vi "CRYProject Editor Global.vi"() -> ()   [LabVIEW 2013]
uses:
  CRYSystem/Typedef Control/CRYTS.ctl
  CRYSystem/Typedef Control/CRYStep.ctl
  CRYSystem/Typedef Control/CRYProjectViewCluster.ctl
  CRYSystem/Typedef Control/CRYHardware.ctl
  CRYSystem/Typedef Control/CRYHardware Channel Info.ctl
panel:
  in  "bProjectLoading Failed":bool
  in  "SubSequenceLanguage":T1(ring)
  in  "SequenceInsertTreeIndex":i32
  in  "SequenceInsert":bool
  in  "G_Calibration Step path":path
  in  "G_Audi Interface Step path":path
  in  "SoundCard Step Backup":T2={"No.VI"=0, "Category"="", "StepName"="", "Seq setup flattened"="", "Comment"="", "Steps config."=[], "Jump config"=[], "Start"=0.0, "Increment"=0.0, "Name"="Pa", "Unit"="Pa", "Y data"=1, "Y prefix"="", "Y dB ref"=1.0, "Y unit"="", "Repeat State Array"=[]} {"Repeat State Array"."Start" format="%#_5g"; "Y dB ref" format="%.1f"; "Y data" items=["dB", "Lin"]; "Start" format="%#_5g"}
  in  "Calibration Step Backup":T2={"No.VI"=0, "Category"="", "StepName"="", "Seq setup flattened"="", "Comment"="", "Steps config."=[], "Jump config"=[], "Start"=0.0, "Increment"=0.0, "Name"="Pa", "Unit"="Pa", "Y data"=1, "Y prefix"="", "Y dB ref"=1.0, "Y unit"="", "Repeat State Array"=[]} {"Repeat State Array"."Start" format="%#_5g"; "Y dB ref" format="%.1f"; "Y data" items=["dB", "Lin"]; "Start" format="%#_5g"}
  in  "Calibration Step VI No":i32
  in  "SoundCard Step VI No":i32
  in  "SoundCard":T3={"Name"="", "Analog I/O"=0, "Digital I/O"=0, "Channels"=2, "Dig Dev ID"=1, "N ports"=3, "Interface"=0, "Dig I/O Ports"=[{"port #"=1, "width"=8, "direction"=0}, {"port #"=2, "width"=8, "direction"=0}, {"port #"=3, "width"=8, "direction"=0}], "Interf settings"=[], "N interfs"=3, "udev SNs"=[], "udev enable"=FALSE, "Channel Array"=[], "Cal sequence"="", "SelectedIn"=0, "SelectedOut"=0, "SelectedTab"=0, "State"=FALSE, "Help"="", "Advanced"=FALSE, "In Audio Driver"=0, "Out Audio Driver"=0} {"Channel Array"."Coupling" items=["Default"=-1, "RSE"=10083, "NRSE"=10078, "Differential"=10106, "Pseudodifferential"=12529]; "Channel Array"."term config" items=["Default"=-1, "RSE"=10083, "NRSE"=10078, "Differential"=10106, "Pseudodifferential"=12529]; "Channel Array"."Anti-aliasing Factor (%fs)" format="%.2f"}
  in  "Calibration Step":T2={"No.VI"=0, "Category"="", "StepName"="", "Seq setup flattened"="", "Comment"="", "Steps config."=[], "Jump config"=[], "Start"=0.0, "Increment"=0.0, "Name"="Pa", "Unit"="Pa", "Y data"=1, "Y prefix"="", "Y dB ref"=1.0, "Y unit"="", "Repeat State Array"=[]} {"Repeat State Array"."Start" format="%#_5g"; "Y dB ref" format="%.1f"; "Y data" items=["dB", "Lin"]; "Start" format="%#_5g"}
  in  "SoundCard Step":T2={"No.VI"=0, "Category"="", "StepName"="", "Seq setup flattened"="", "Comment"="", "Steps config."=[], "Jump config"=[], "Start"=0.0, "Increment"=0.0, "Name"="Pa", "Unit"="Pa", "Y data"=1, "Y prefix"="", "Y dB ref"=1.0, "Y unit"="", "Repeat State Array"=[]} {"Repeat State Array"."Start" format="%#_5g"; "Y dB ref" format="%.1f"; "Y data" items=["dB", "Lin"]; "Start" format="%#_5g"}
  in  "Add Step":refnum<vi>
  in  "Expand/Collapse Btn":refnum<vi>
  in  "TS Tree1":refnum<vi>
  in  "Property seq":refnum<vi>
  in  "Property step":refnum<vi>
  in  "Remove":refnum<vi>
  in  "Move Up":refnum<vi>
  in  "Move Down":refnum<vi>
  in  "TS Name":refnum<vi>
  in  "Expand/Collapse":bool
  in  "ConfigureShow":bool
  in  "Sequence Index for Calibration":i32
  in  "Sequence Index for Hardware":i32
  in  "ProjectViewCluster Array":T5[](array[typedef])
  in  "bProjectChanged":bool
  in  "bProjectLoaded":bool
  in  "cMsgProject":T6
  in  "previous cursor ID":refnum<k1>
  in  "sWorkAction":string
  in  "New Sequence Number":u16
  in  "PathLog":path
  in  "TS Array":T7 {"Steps"."Repeat State Array"."Start" format="%#_5g"; "Steps"."Y dB ref" format="%.1f"; "Steps"."Y data" items=["dB", "Lin"]; "Steps"."Start" format="%#_5g"}
  in  "Display Step No":i32
  in  "Project Open Mode":bool
  in  "Project Exist?":bool
  in  "ExitStateVal":u8
  in  "ScrollStateFlg":bool
  in  "ScrollStateVal":u8
  in  "Calibration TS Array":T7 {"Steps"."Repeat State Array"."Start" format="%#_5g"; "Steps"."Y dB ref" format="%.1f"; "Steps"."Y data" items=["dB", "Lin"]; "Steps"."Start" format="%#_5g"}
  in  "step ID Max":i16
  in  "TS Edit Info":cluster{"In Channel":u16, "Out Channel":u16}
  in  "AddStepsVI":refnum<vi>
  in  "ProjectView VI":refnum<vi>
  in  "AddStepCluster":T8
  in  "Task Sequence NameRef":refnum<vi>
  in  "Default TS Name":string
  in  "AddStepContent":T9(array[cluster])
  in  "SelectTreeStepNumber":i32
  in  "Step Setup VI No":i32
  # "Curves Array"
  # "max value"
  # "Selected Curves Array"
  # "old step edit num"
  # "current edit step"
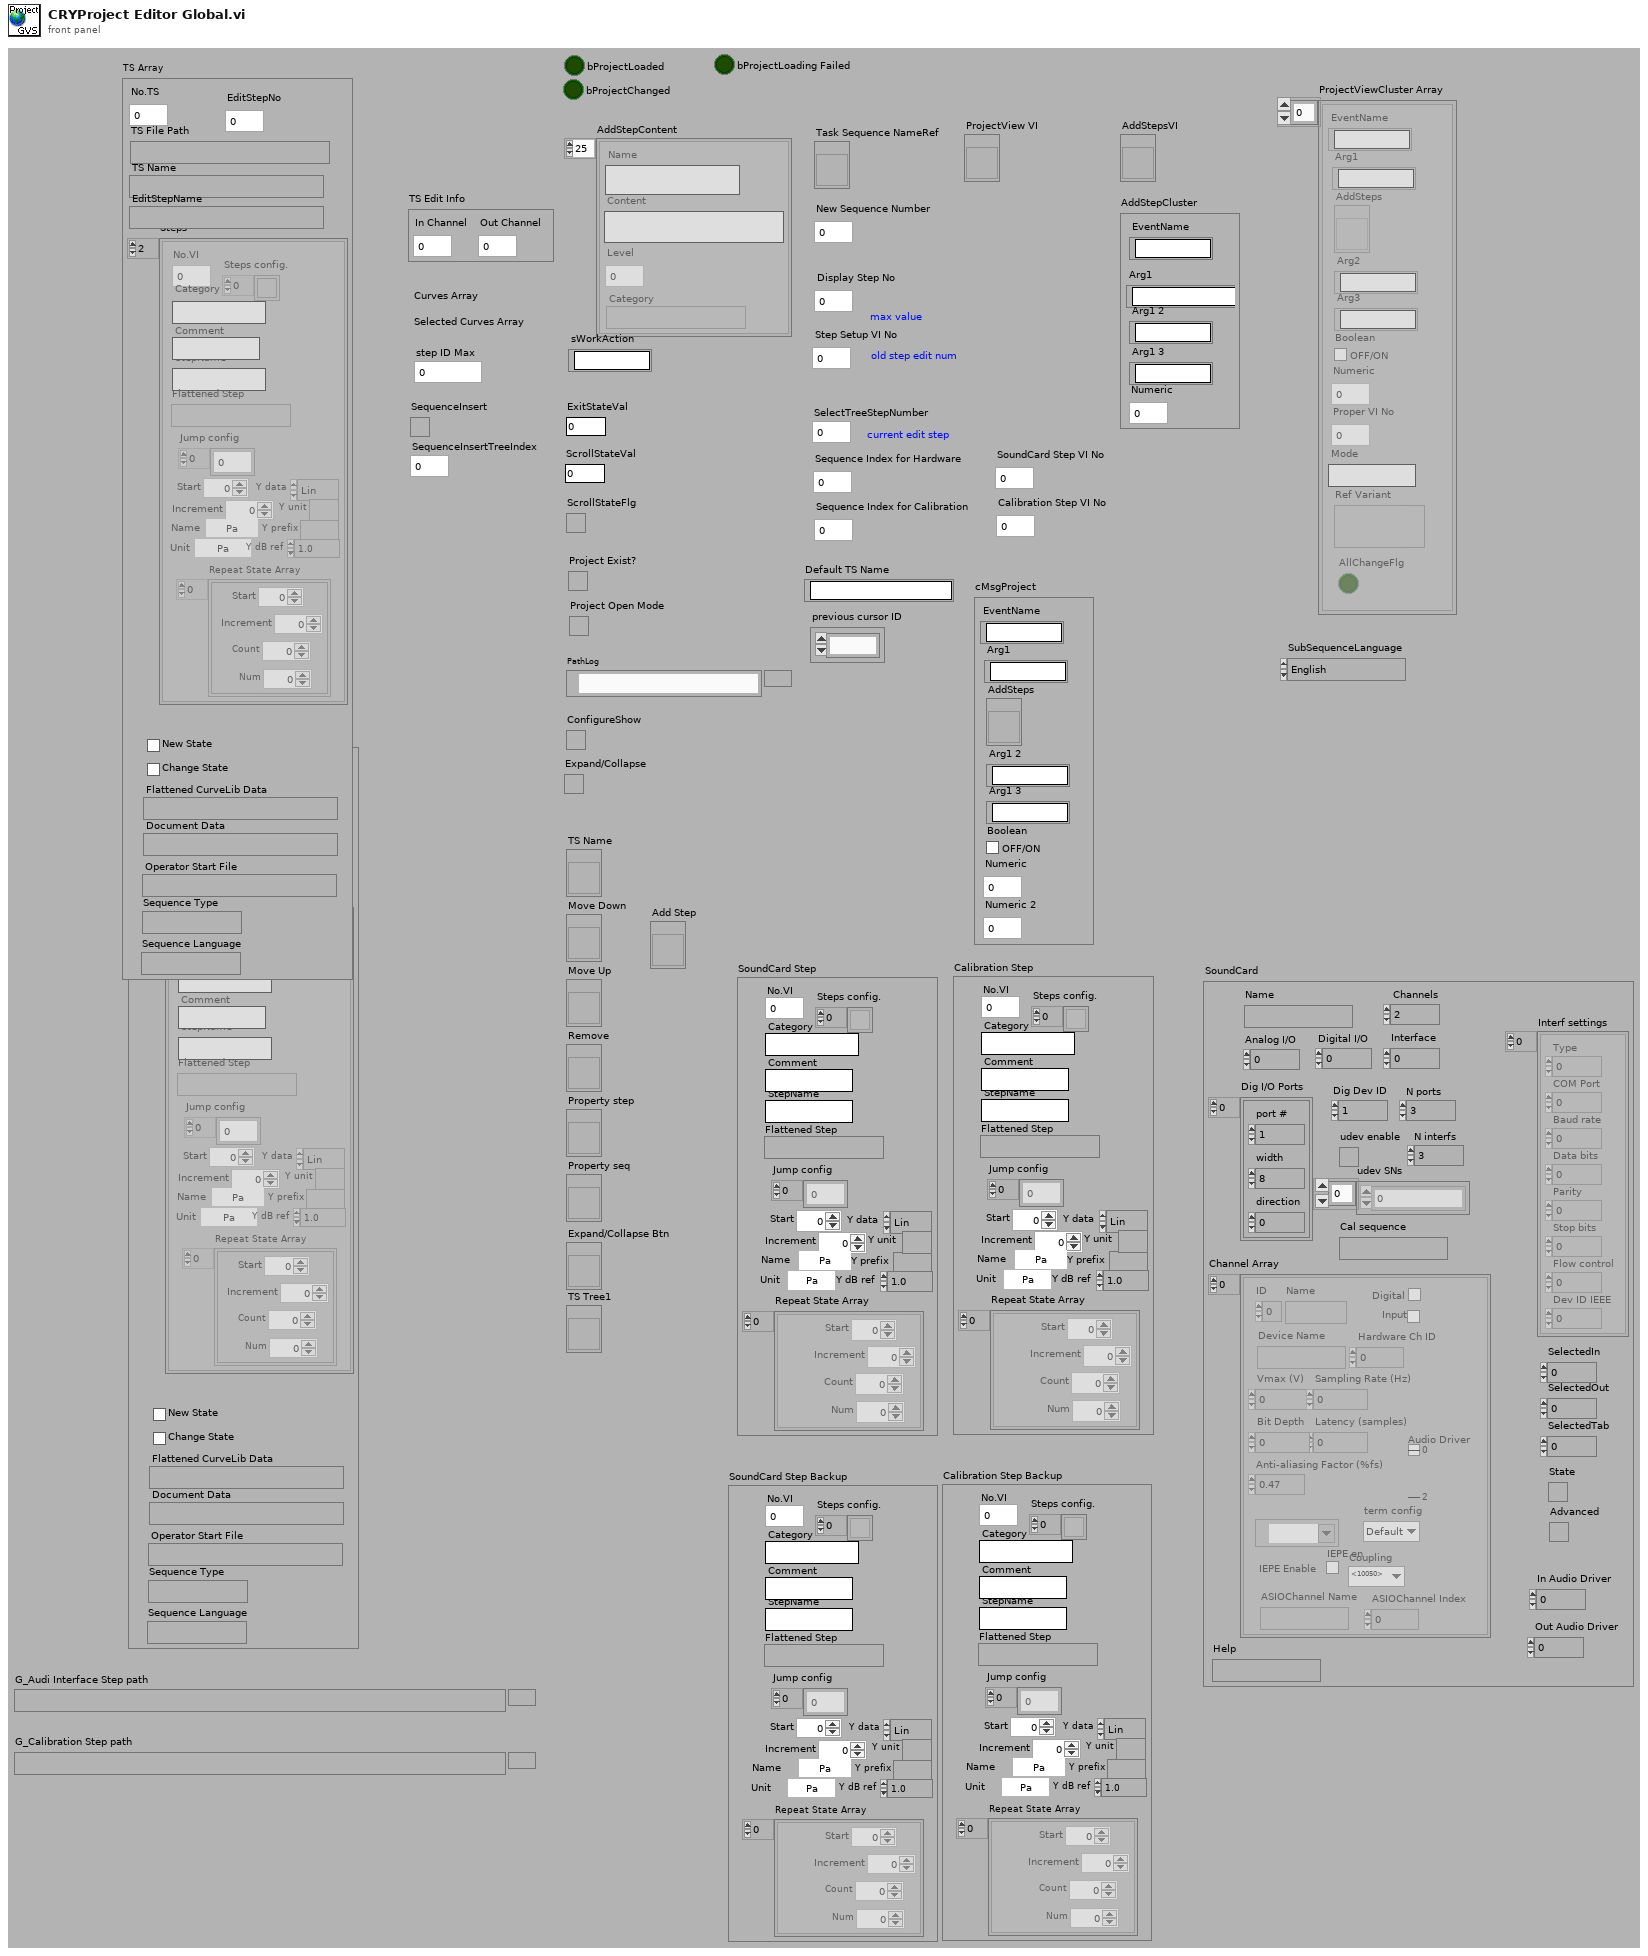
[diagram p1: front panel]
types:
  T1 = enum32{"English", "Chinese", "Korean", "Japanese", "Russian", "Chinese traditional"}
  T2 = typedef "CRYStep.ctl" = cluster{"No.VI":i32, "Category":string, "StepName":string, "Seq setup flattened":string, "Comment":string, "Steps config.":bool[], "Jump config":i32[], "Start":dbl, "Increment":dbl, "Name":string, "Unit":string, "Y data":u16, "Y prefix":string, "Y dB ref":dbl, "Y unit":string, "Repeat State Array":cluster{"Start":dbl, "Increment":dbl, "Count":i32, "Num":i32}[]}
  T3 = typedef "CRYHardware.ctl" = cluster{"Name":string, "Analog I/O":u16, "Digital I/O":u16, "Channels":u8, "Dig Dev ID":u8, "N ports":u8, "Interface":u32, "Dig I/O Ports":cluster{"port #":i16, "width":i16, "direction":i32}[], "Interf settings":cluster{"Type":u16, "COM Port":u8, "Baud rate":u32, "Data bits":u32, "Parity":u16, "Stop bits":u16, "Flow control":u16, "Dev ID IEEE":u8}[], "N interfs":i32, "udev SNs":i16[], "udev enable":bool, "Channel Array":T4[], "Cal sequence":string, "SelectedIn":u16, "SelectedOut":u16, "SelectedTab":u16, "State":bool, "Help":string, "Advanced":bool, "In Audio Driver":u16, "Out Audio Driver":u16}
  T4 = typedef "CRYHardware Channel Info.ctl" = cluster{"ID":i32, "Name":string, "Digital":bool, "Input":bool, "Device Name":string, "Hardware Ch ID":u8, "Vmax (V)":dbl, "Latency (samples)":dbl, "Sampling Rate (Hz)":u32, "Bit Depth":u32, "Anti-aliasing Factor (%fs)":sgl, "DAQmx Channel":tag, "term config":i32, "Coupling":i32, "IEPE en":bool, "ASIOChannel Name":string, "Audio Driver":u16, "ASIOChannel Index":u8}
  T5 = typedef "CRYProjectViewCluster.ctl" = cluster{"EventName":string, "Arg1":string, "Numeric":i32, "Proper VI No":i32, "AddSteps ":refnum<vi>, "Arg2":string, "Arg3":string, "Boolean":bool, "Mode":string, "Ref Variant":variant, "AllChangeFlg":bool}
  T6 = cluster{"EventName":string, "Arg1":string, "Numeric":u16, "Numeric 2":u16, "AddSteps ":refnum<vi>, "Arg1 2":string, "Arg1 3":string, "Boolean":bool}
  T7 = typedef "CRYTS.ctl" = cluster{"No.TS":u16, "TS File Path":path, "TS Name":string, "EditStepName":string, "Steps":T2[], "New State":bool, "Change State":bool, "Flattened CurveLib Data":string, "Document Data":string, "EditStepNo":u16, "Operator Start File":string, "Sequence Type":string, "Sequence Language":string}
  T8 = cluster{"EventName":string, "Arg1":string, "Arg1 2":string, "Numeric":dbl, "Arg1 3":string}
  T9 = cluster{"Content":string, "Name":string, "Level":u32, "Category":string}[]
diagram:
